vi "Close.vi"(8 "error in (no error)":errorcluster, 11 "INI Deserializer in":refnum<class "INI Deserializer.lvclass">) -> (0 "error out":errorcluster)   [LabVIEW 2014, in "INI Deserializer.lvclass"]
uses:
  INI Deserializer.lvclass
  INI Deserializer.lvclass/INI Deserializer.ctl
  <vilib>/Utility/config.llb/NI_LVConfig.lvlib
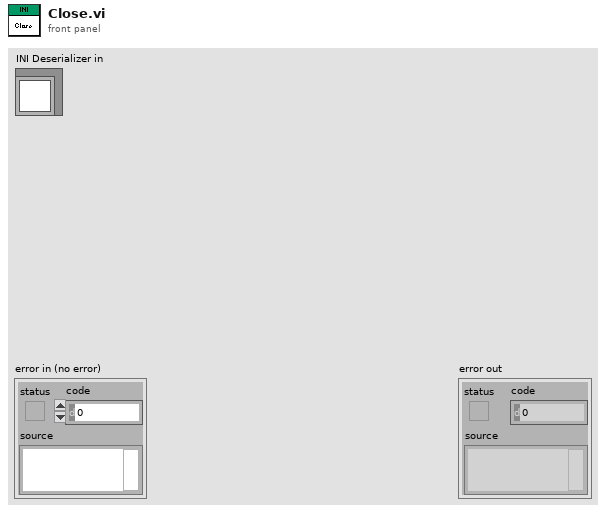
[diagram p1: front panel]
types:
  T1 = typedef "NI_LVConfig.lvlib/Config Data RefNum.ctl" = refnum<k1>
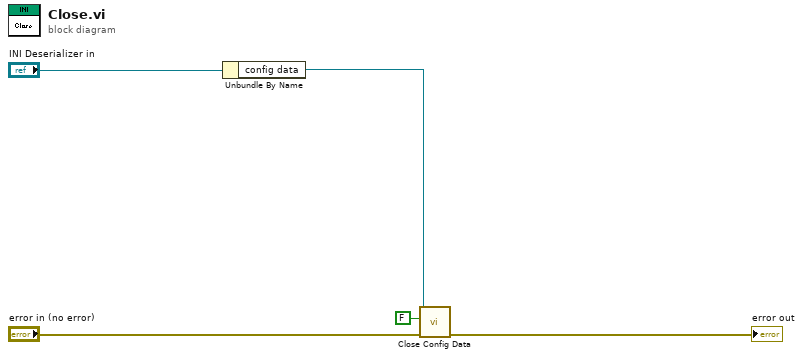
[diagram p0: block diagram]
diagram:
  n1 = Unbundle By Name("INI Deserializer in") -> ("config data"=w5:T1)
  n2 = call <vilib>:"Close Config Data.vi"("error in (no error)"="error in (no error)", "write file if changed (T)"=FALSE, "refnum"=w5) -> ("error out"=→"error out":errorcluster)  [unwired: 7 in, 1 out]
